vi "ServoSmartTurn.vi"(8 "error in":errorcluster, 9 "Turn to (in)":T1, 11 "Servo":T2) -> (0 "error out":errorcluster, 3 "Turn State (out)":T1)   [LabVIEW 2017, in "RubikLibrary.lvlib"]
doc: "Servo turning VI. \nThree turning servos allowed (Left, Front,Right).\nAbsolute angular positions +/-90° and 0°.\n\n1) Configure PWM frequency, conversion from degrees to duty cycle\n2) Assign PWM A channels to servo\n3) (Smart) Open PWM A channel\n4) Move servo, turn to angular positions +90°,0°,-90°\n\nReturns the final position, so that state might be maintained. \n\nExecution type: Preallocated clone reentrant execution\nThe addition of the case structure is necessary to keep the correct status (channel). Otherwise the status of the VI does not correlate to the corresponding servo. Each servo (hardware) demands its own VI (software)."
uses:
  RubikLibrary.lvlib
  ServoAbsAngleControl.ctl
  ServoEnumControl.ctl
  <vilib>/Utility/error.llb/Error Cluster From Error Code.vi
  <vilib>/myRIO/Common/Instrument Driver Framework/myRIO v1.0/PWM/vis/myRIO v1.0 Write PWM.vi
  <vilib>/myRIO/Instrument Drivers/Onboard IO/PWM/PWM.lvlib
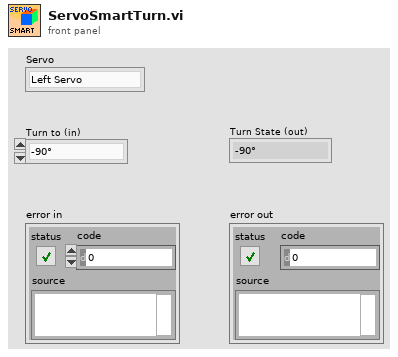
[diagram p1: front panel]
types:
  T1 = typedef "RubikLibrary.lvlib/ServoAbsAngleControl.ctl" = enum16{"-90°", "0°", "+90°"}
  T2 = typedef "RubikLibrary.lvlib/ServoEnumControl.ctl" = enum16{"Left Servo", "Front Servo", "Right Servo"}
  T3 = typedef "PWM.lvlib/PWM Reference.ctl" = cluster{"myRIO Reference":T4, "PWM Channels Enum":T8, "PWM Configuration":T9}
  T4 = typedef "myRIO Generic Hardware Reference.ctl" = cluster{"myRIO Model":T5, "myRIO Hardware Reference":T6}
  T5 = typedef "Hardware Version Enum.ctl" = enum16{"Unknown", "myRIO-1900", "myRIO-1950", "roboRIO", "NI ELVIS RIO CM"}
  T6 = typedef "myRIO v1.0 Reference.ctl" = cluster{"Generic FPGA Reference":T7, "Allow multiple opens":bool}
  T7 = typedef "Generic FPGA Reference.ctl" = refnum<k20>
  T8 = typedef "PWM Channels Enum.ctl" = enum16{"Not Connected", "C/PWM0", "C/PWM1", "A/PWM0", "A/PWM1", "A/PWM2", "B/PWM0", "B/PWM1", "B/PWM2", "PWM/PWM0", "PWM/PWM1", "PWM/PWM2", "PWM/PWM3", "PWM/PWM4", "PWM/PWM5", "PWM/PWM6", "PWM/PWM7", "PWM/PWM8", "PWM/PWM9"}
  T9 = typedef "PWM.lvlib/PWM Configuration.ctl" = cluster{"Frequency":dbl, "Duty Cycle":dbl}
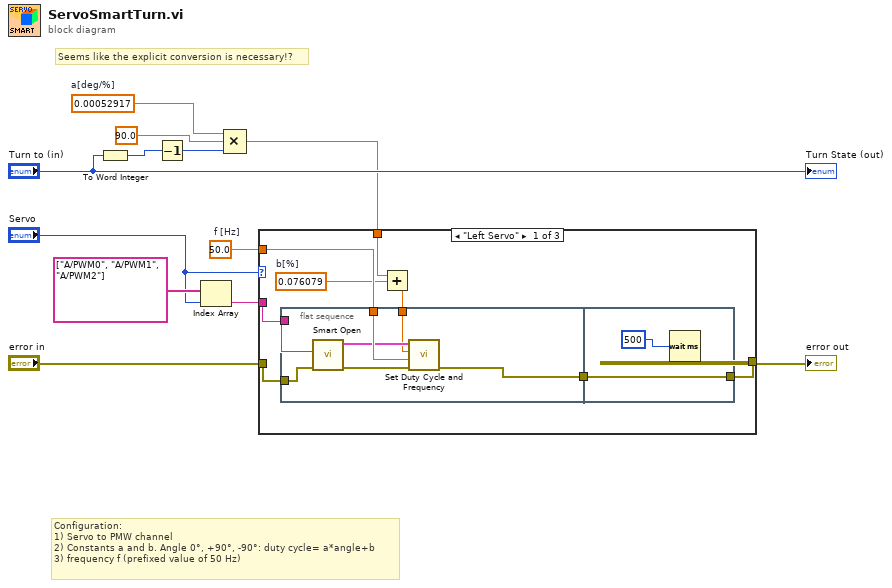
[diagram p0: block diagram]
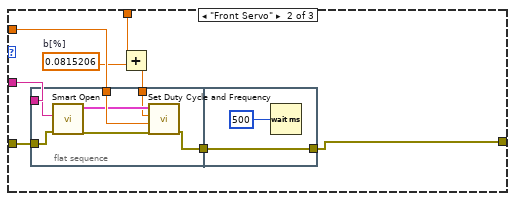
[diagram p2: hidden frame]
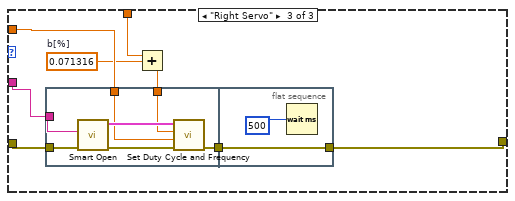
[diagram p3: hidden frame]
diagram:
  w4 = 0.00052917  # a[deg/%]
  w12 = 50.0  # f [Hz]
  # "Seems like the explicit conversion is necessary!?"
  # "Configuration:\n1) Servo to PMW channel\n2) Constants a and b. Angle 0°, +90°, -90°: duty cycle= a*angle+b\n3) frequency f (prefixed value of 50 Hz)"
  n1 = To Word Integer(number="Turn to (in)") -> (16bit integer=w5:i16)
  n2 = Decrement(x=w5) -> (x-1=w2:i16)
  n3 = Index Array(array=tag[] ["A/PWM0", "A/PWM1", "A/PWM2"], index="Servo") -> (element=w8:tag)
  n4 = Compound Arithmetic op=MULTIPLY(w4, 90.0, w2) -> (w1:dbl)
  n5 = case shown="\"Left Servo\"" "Servo" {
    tunnel: w12 -> [w20 w37 w51]
    tunnel: "error in" -> [w18 w36 w53]
    tunnel: [w19 w33 w54] -> w10
    tunnel: w8 -> [w17 w35 w52]
    tunnel: w1 -> [w14 w31 w49]
    frame "Left Servo" {
      w15 = 0.076079  # b[%]
      n6 = flat-sequence {
        tunnel: w20 -> [w26]
        tunnel: w18 -> [w24]
        tunnel: w17 -> [w23]
        tunnel: [w25] -> w16
        tunnel: w13 -> [w21]
        tunnel: [w29] -> w19
        tunnel: w16 -> [w29]
        frame #0 {
          n7 = call <vilib>:"Smart Open.vi"("error in (no error)"=w24, "Channel Name"=w23) -> ("error out"=w27:errorcluster, "PWM Ref Out"=w22:T3)  [unwired: 8 in]
          n8 = call <vilib>:"Set Duty Cycle and Frequency.vi"("error in (no error)"=w27, "Frequency [Hz]"=w26, "Duty Cycle"=w21, "PWM Ref In"=w22) -> ("error out"=w25:errorcluster)  [unwired: 5 in, 1 out]
        }
        frame #1 {
          n9 = Wait (ms)(milliseconds to wait=u32 500) -> ()  [unwired: 1 out]
        }
      }
      n10 = Add(x=w14, y=w15) -> (x+y=w13:dbl)
    }
    frame "Front Servo" {
      w32 = 0.0815206  # b[%]
      n11 = flat-sequence {
        tunnel: w37 -> [w44]
        tunnel: w36 -> [w43]
        tunnel: w35 -> [w39]
        tunnel: [w40] -> w34
        tunnel: w30 -> [w38]
        tunnel: [w46] -> w33
        tunnel: w34 -> [w46]
        frame #0 {
          n12 = call <vilib>:"Smart Open.vi"("error in (no error)"=w43, "Channel Name"=w39) -> ("error out"=w41:errorcluster, "PWM Ref Out"=w42:T3)  [unwired: 8 in]
          n13 = call <vilib>:"Set Duty Cycle and Frequency.vi"("error in (no error)"=w41, "Frequency [Hz]"=w44, "Duty Cycle"=w38, "PWM Ref In"=w42) -> ("error out"=w40:errorcluster)  [unwired: 5 in, 1 out]
        }
        frame #1 {
          n14 = Wait (ms)(milliseconds to wait=u32 500) -> ()  [unwired: 1 out]
        }
      }
      n15 = Add(x=w31, y=w32) -> (x+y=w30:dbl)
    }
    frame "Right Servo" {
      w48 = 0.071316  # b[%]
      n16 = flat-sequence {
        tunnel: w53 -> [w58]
        tunnel: w52 -> [w57]
        tunnel: w51 -> [w56]
        tunnel: [w59] -> w50
        tunnel: w47 -> [w55]
        tunnel: [w63] -> w54
        tunnel: w50 -> [w63]
        frame #0 {
          n17 = call <vilib>:"Smart Open.vi"("error in (no error)"=w58, "Channel Name"=w57) -> ("error out"=w61:errorcluster, "PWM Ref Out"=w60:T3)  [unwired: 8 in]
          n18 = call <vilib>:"Set Duty Cycle and Frequency.vi"("error in (no error)"=w61, "Frequency [Hz]"=w56, "Duty Cycle"=w55, "PWM Ref In"=w60) -> ("error out"=w59:errorcluster)  [unwired: 5 in, 1 out]
        }
        frame #1 {
          n19 = Wait (ms)(milliseconds to wait=u32 500) -> ()  [unwired: 1 out]
        }
      }
      n20 = Add(x=w49, y=w48) -> (x+y=w47:dbl)
    }
  }
  "error out" <- w10
  "Turn State (out)" <- "Turn to (in)"
